vi "Problem2.2.vi"() -> ()   [LabVIEW 2019]
panel:
  out "Timer Done":bool
  in  "Wait Time (Seconds)":dbl=4.0
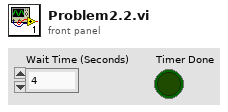
[diagram p1: front panel]
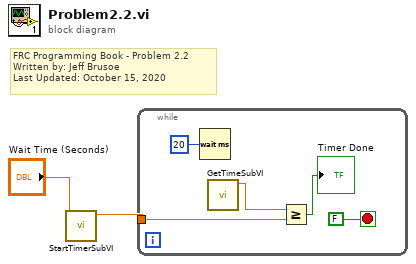
[diagram p0: block diagram]
diagram:
  # "FRC Programming Book - Problem 2.2\nWritten by: Jeff Brusoe\nLast Updated: October 15, 2020"
  n1 = call "StartTimerSubVI.vi"("Wait Time (Seconds)"="Wait Time (Seconds)") -> ("End Time (Seconds)"=w1:dbl)  [unwired: 10 in]
  n2 = while {
    tunnel: w1 -> [w4]
    stop <- FALSE stop-if-true
    n3 = Wait (ms)(milliseconds to wait=u32 20) -> ()  [unwired: 1 out]
    n4 = call "GetTimeSubVI.vi"() -> ("Seconds"=w3:dbl)  [unwired: 11 in]
    n5 = Greater Or Equal?(x=w3, y=w4) -> (x >= y?=→"Timer Done":bool)
  }
